vi "Initialize.vi"(8 "error in (no error)":errorcluster, 10 "DAQ Class.lvclass":refnum<class "DAQ Class.lvclass">, 11 "Intensity Processing in":refnum<class "Intensity Processing.lvclass">) -> (0 "error out":errorcluster, 3 "Intensity Processing out":refnum<class "Intensity Processing.lvclass">)   [LabVIEW 2014, in "Intensity Processing.lvclass"]
uses:
  Intensity Processing.lvclass
  Classes/DAQ/DAQ Class.lvclass
  Classes/Processing.lvclass
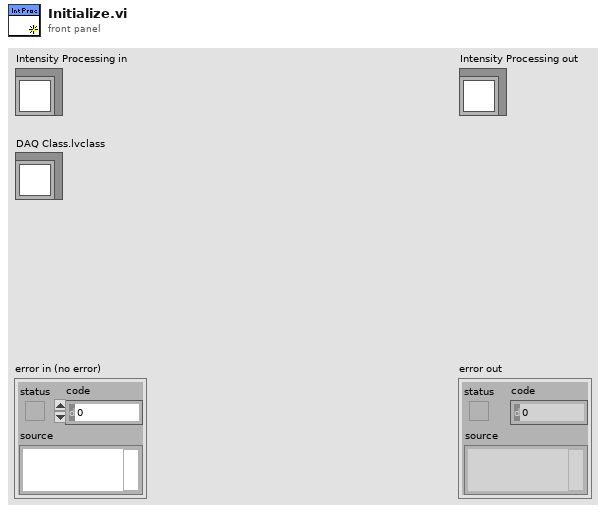
[diagram p1: front panel]
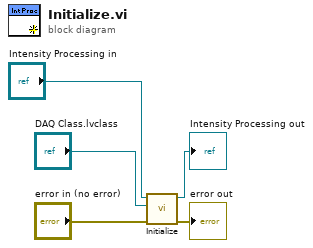
[diagram p0: block diagram]
diagram:
  n1 = call-parent "Initialize.vi"("error in (no error)"="error in (no error)", "DAQ Class.lvclass"="DAQ Class.lvclass", "Processing in"="Intensity Processing in") -> ("error out"=→"error out":errorcluster, "Processing out"=→"Intensity Processing out":refnum<class "Intensity Processing.lvclass">)  [unwired: 7 in]
